vi "test log.vi"() -> ()   [LabVIEW 2010]
uses:
  DLL-s/MakeFullImmitationStepDLL/Release/MakeFullImmitationStepDLL.dll
panel:
  out "return type":i32
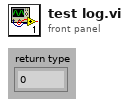
[diagram p1: front panel]
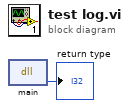
[diagram p0: block diagram]
diagram:
  n1 = dll-call lib="D:/Liakh Tanya/Dissertation/Complex/DLL-s/MakeFullImmitationStepDLL/Release/MakeFullImmitationStepDLL.dll" fn="main"() -> ("return type"=→"return type":i32)  [unwired: 3 in, 2 out]
